vi "PCO_SetColorSettings.vi"(8 "error in (no error)":errorcluster {"code" format="%x"}, 10 "strColorSet":T1, 11 "ph":u64) -> (0 "error out":errorcluster {"code" format="%x"}, 2 "ErrorMessage":i32 format="%x", 3 "ph out":u64)   [LabVIEW 2020, in "SDK.lvlib" / "SpecialCommandsDimax_HDSDI.lvlib"]
doc: "<b>Description:</b>\nSets the color convert parameters of the camera.\n\n<b>Supported camera type:</b>\npco.dimax with HD-SDI interface\n\n<b>Descriptor dependency:</b>\nNone"
uses:
  SpecialCommandsDimax_HDSDI.lvlib
  Structures.lvlib
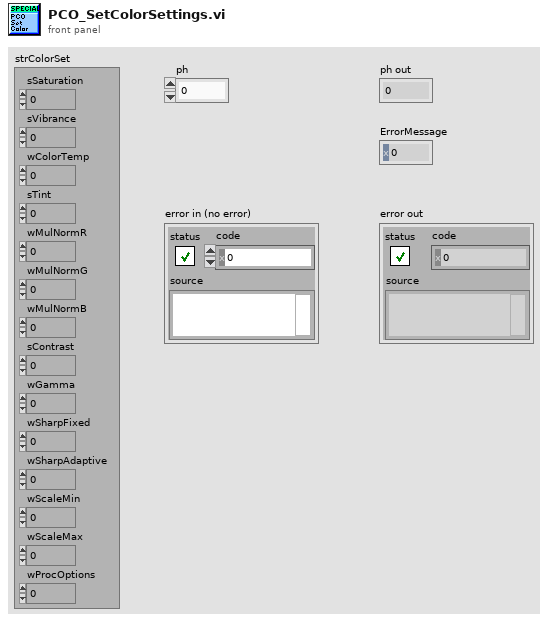
[diagram p1: front panel]
types:
  T1 = cluster{"sSaturation":i16, "sVibrance":i16, "wColorTemp":u16, "sTint":i16, "wMulNormR":u16, "wMulNormG":u16, "wMulNormB":u16, "sContrast":i16, "wGamma":u16, "wSharpFixed":u16, "wSharpAdaptive":u16, "wScaleMin":u16, "wScaleMax":u16, "wProcOptions":u16}
  T2 = cluster{"wSize":u16, "sSaturation":i16, "sVibrance":i16, "wColorTemp":u16, "sTint":i16, "wMulNormR":u16, "wMulNormG":u16, "wMulNormB":u16, "sContrast":i16, "wGamma":u16, "wSharpFixed":u16, "wSharpAdaptive":u16, "wScaleMin":u16, "wScaleMax":u16, "wProcOptions":u16, "ZZwDummy":cluster{u16, u16, u16, u16, u16, u16, u16, u16, u16, u16, u16, u16, u16, u16, u16, u16, u16, u16, u16, u16, u16, u16, u16, u16, u16, u16, u16, u16, u16, u16, u16, u16, u16, u16, u16, u16, u16, u16, u16, u16, u16, u16, u16, u16, u16, u16, u16, u16, u16, u16, u16, u16, u16, u16, u16, u16, u16, u16, u16, u16, u16, u16, u16, u16, u16, u16, u16, u16, u16, u16, u16, u16, u16, u16, u16, u16, u16, u16, u16, u16, u16, u16, u16, u16, u16, u16, u16, u16, u16, u16, u16, u16, u16}}
  T3 = cluster{u16, u16, u16, u16, u16, u16, u16, u16, u16, u16, u16, u16, u16, u16, u16, u16, u16, u16, u16, u16, u16, u16, u16, u16, u16, u16, u16, u16, u16, u16, u16, u16, u16, u16, u16, u16, u16, u16, u16, u16, u16, u16, u16, u16, u16, u16, u16, u16, u16, u16, u16, u16, u16, u16, u16, u16, u16, u16, u16, u16, u16, u16, u16, u16, u16, u16, u16, u16, u16, u16, u16, u16, u16, u16, u16, u16, u16, u16, u16, u16, u16, u16, u16, u16, u16, u16, u16, u16, u16, u16, u16, u16, u16}
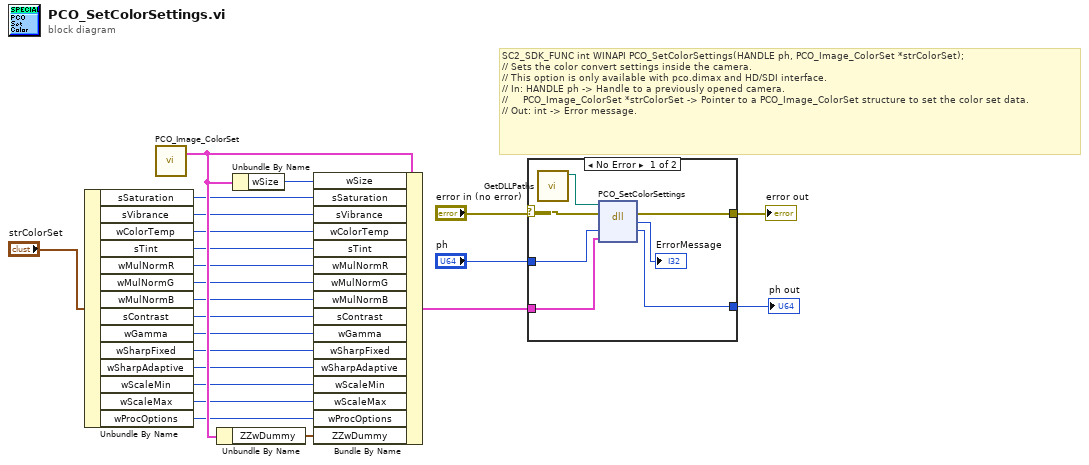
[diagram p0: block diagram]
diagram:
  # "SC2_SDK_FUNC int WINAPI PCO_SetColorSettings(HANDLE ph, PCO_Image_ColorSet *strColorSet);\n// Sets the color convert settings inside the camera.\n// This option is only available with pco.dimax and HD/SDI interface.\n// In: HANDLE ph -> Handle to a previously opened camera.\n//     PCO_Image_ColorSet *strColorSet -> Pointer to a PCO_Image_ColorSet structure to set the color set data.\n// Out: int -> Error message."
  n1 = Unbundle By Name("strColorSet") -> ("sSaturation"=w15:i16, "sVibrance"=w14:i16, "wColorTemp"=w13:u16, "sTint"=w12:i16, "wMulNormR"=w11:u16, "wMulNormG"=w10:u16, "wMulNormB"=w9:u16, "sContrast"=w8:i16, "wGamma"=w7:u16, "wSharpFixed"=w6:u16, "wSharpAdaptive"=w5:u16, "wScaleMin"=w4:u16, "wScaleMax"=w3:u16, "wProcOptions"=w2:u16)
  n2 = call "PCO_Image_ColorSet.vi"() -> ("PCO_Image_ColorSet_Raw"=w17:T2)  [unwired: 4 in, 3 out]
  n3 = Unbundle By Name(w17) -> ("ZZwDummy"=w16:T3)
  n4 = Unbundle By Name(w17) -> ("wSize"=w18:u16)
  n5 = Bundle By Name(cluster=w17, "wSize"=w18, "sSaturation"=w15, "sVibrance"=w14, "wColorTemp"=w13, "sTint"=w12, "wMulNormR"=w11, "wMulNormG"=w10, "wMulNormB"=w9, "sContrast"=w8, "wGamma"=w7, "wSharpFixed"=w6, "wSharpAdaptive"=w5, "wScaleMin"=w4, "wScaleMax"=w3, "wProcOptions"=w2, "ZZwDummy"=w16) -> (w1:T2)
  n6 = case shown="No Error" "error in (no error)" {
    selector: "error in (no error)" -> [w25 w32]
    tunnel: "ph" -> [w29 w31]
    tunnel: [w28 w31] -> w22
    tunnel: w1 -> [w27 _]
    tunnel: [w26 w32] -> w21
    frame No Error {
      n7 = call "GetDLLPaths.vi"() -> ("SC2_Cam_Path"=w24:path)  [unwired: 9 in, 2 out]
      n8 = dll-call lib="?" fn="PCO_SetColorSettings"(path in=w24, error in=w25, "ph"=w29, "strColorSet"=w27) -> (error out=w26:errorcluster, "return type"=→"ErrorMessage":i32, "ph"=w28:u64)  [unwired: 2 in, 1 out]
    }
    frame Error {
    }
  }
  "ph out" <- w22
  "error out" <- w21
